vi "Calculate PWM.vi"(10 "Value":T1 {"Air Pump PWM" min=0 max=99.9 step=0.1 scale=0.0..100.0}, 11 "Pump Flow Rate":u16) -> (3 "PWM":dbl)   [LabVIEW 2016]
uses:
  Controls/AirPump Controls.ctl
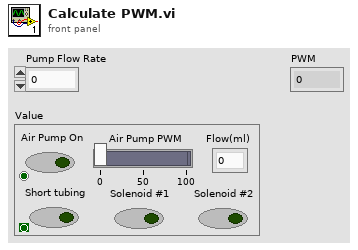
[diagram p1: front panel]
types:
  T1 = typedef "AirPump Controls.ctl" = cluster{"Air Pump PWM":sgl, "Solenoid #1":bool, "Solenoid #2":bool, "Air Pump On":bool, "Short tubing":bool, "Loflo Connected":bool, "Flow(ml)":u16, "Wait Active":bool}
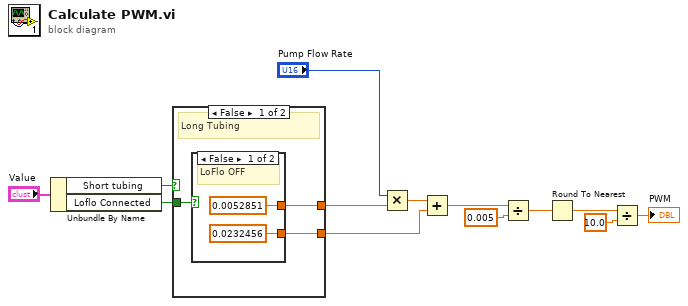
[diagram p0: block diagram]
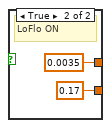
[diagram p2: hidden frame]
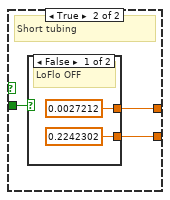
[diagram p3: hidden frame]
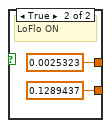
[diagram p4: hidden frame]
diagram:
  n1 = Unbundle By Name("Value") -> ("Short tubing"=w12:bool, "Loflo Connected"=w13:bool)
  n2 = case shown="False" w12 {
    tunnel: w13 -> [w14 w21]
    tunnel: [w15 w23] -> w1
    tunnel: [w16 w22] -> w2
    frame False {
      # "Long Tubing"
      n3 = case shown="False" w14 {
        tunnel: [0.0232456 0.17] -> w15
        tunnel: [0.0052851 0.0035] -> w16
        frame False {
          # "LoFlo OFF"
        }
        frame True {
          # "LoFlo ON"
        }
      }
    }
    frame True {
      # "Short tubing"
      n4 = case shown="False" w21 {
        tunnel: [0.2242302 0.1289437] -> w23
        tunnel: [0.0027212 0.0025323] -> w22
        frame False {
          # "LoFlo OFF"
        }
        frame True {
          # "LoFlo ON"
        }
      }
    }
  }
  n5 = Multiply(x="Pump Flow Rate", y=w2) -> (x*y=w4:dbl)
  n6 = Add(x=w4, y=w1) -> (x+y=w5:dbl)
  n7 = Divide(x=w5, y=0.005) -> (x/y=w7:dbl)
  n8 = Round To Nearest(number=w7) -> (nearest integer value=w9:dbl)
  n9 = Divide(x=w9, y=10.0) -> (x/y=→"PWM":dbl)
